vi "Read Constant Sizes.vi"(8 "error in (no error)":errorcluster, 11 "BetterHandle in":refnum<class "BetterHandle.lvclass">) -> (0 "error out":errorcluster, 2 "constant pixel sizes":T1, 3 "BetterHandle out":refnum<class "BetterHandle.lvclass">)   [LabVIEW 2020, in "BetterDragAndDrop.lvlib" / "BetterHandle.lvclass"]
uses:
  BetterHandle.lvclass
  Pixel Constants.ctl
  BetterHandle.lvclass/BetterHandle.ctl
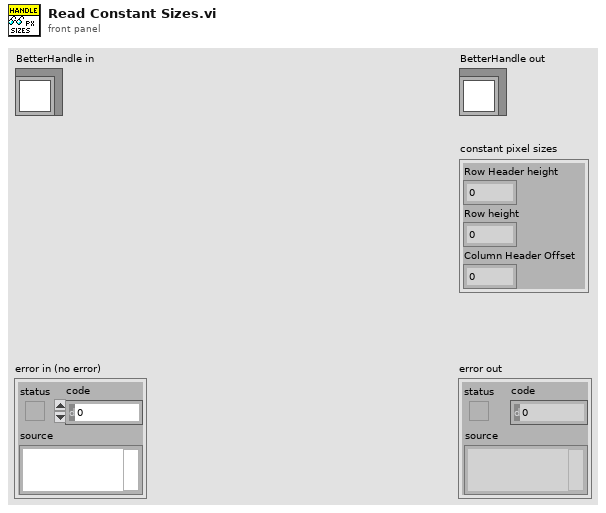
[diagram p1: front panel]
types:
  T1 = typedef "BetterDragAndDrop.lvlib/BetterHandle.lvclass/Pixel Constants.ctl" = cluster{"Row Header height":i32, "Row height":i32, "Column Header Offset":i32}
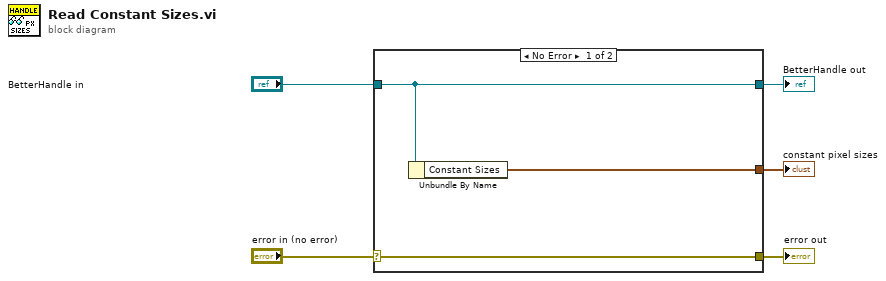
[diagram p0: block diagram]
diagram:
  n1 = case shown="No Error" "error in (no error)" {
    selector: "error in (no error)" -> [w8 w9]
    tunnel: [w8 w9] -> w4
    tunnel: [w7 w10] -> w2
    tunnel: "BetterHandle in" -> [w7 w10]
    tunnel: [w6 _] -> w1
    frame No Error {
      n2 = Unbundle By Name(w7) -> ("Constant Sizes"=w6:T1)
    }
    frame Error {
    }
  }
  "error out" <- w4
  "BetterHandle out" <- w2
  "constant pixel sizes" <- w1
